vi "Cylindrical to Spherical.vi"(4 "Cylindrical\nCoordinates":cluster{"r":dbl, "theta":dbl, "z":dbl}) -> (1 "Spherical\nCoordinates":cluster{"rho":dbl, "theta":dbl, "phi":dbl})   [LabVIEW 2013]
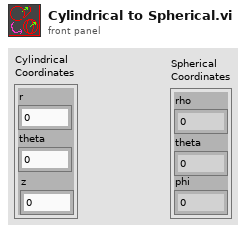
[diagram p1: front panel]
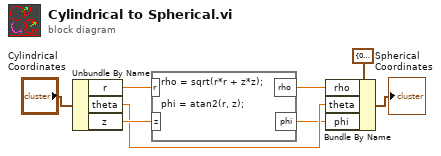
[diagram p0: block diagram]
diagram:
  n1 = Unbundle By Name("Cylindrical\nCoordinates") -> ("r"=w5:dbl, "theta"=w2:dbl, "z"=w4:dbl)
  n2 = formula code="rho = sqrt(r*r + z*z);\n\nphi = atan2(r, z);"("r"=w5, "z"=w4) -> ("rho"=w3:dbl, "phi"=w1:dbl)
  n3 = Bundle By Name(cluster=cluster{"rho":dbl, "theta":dbl, "phi":dbl} {"rho"=0.0, "theta"=0.0, "phi"=0.0} ("input cluster"), "rho"=w3, "theta"=w2, "phi"=w1) -> (→"Spherical\nCoordinates":cluster{"rho":dbl, "theta":dbl, "phi":dbl})
